vi "Write Frame (iSUB) (SubVI).vi"(5 "Data":T1, 8 "Record":bool, 11 "FILE REF IN":refnum<file>) -> (3 "FILE REF OUT":refnum<file>)   [LabVIEW 2015]
uses:
  Controls (HOST)/Data to Disk Bundle.ctl
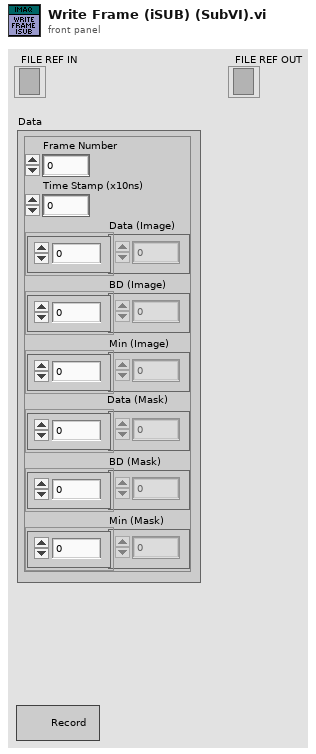
[diagram p1: front panel]
types:
  T1 = typedef "Data to Disk Bundle.ctl" = cluster{"Frame Number":u64, "Time Stamp (x10ns)":u64, "Data (Image)":u64[], "BD (Image)":u8[], "Min (Image)":u8[], "Data (Mask)":u64[], "BD (Mask)":u8[], "Min (Mask)":u8[]}
  T2 = enum16{"big-endian, network order", "native, host order", "little-endian"}
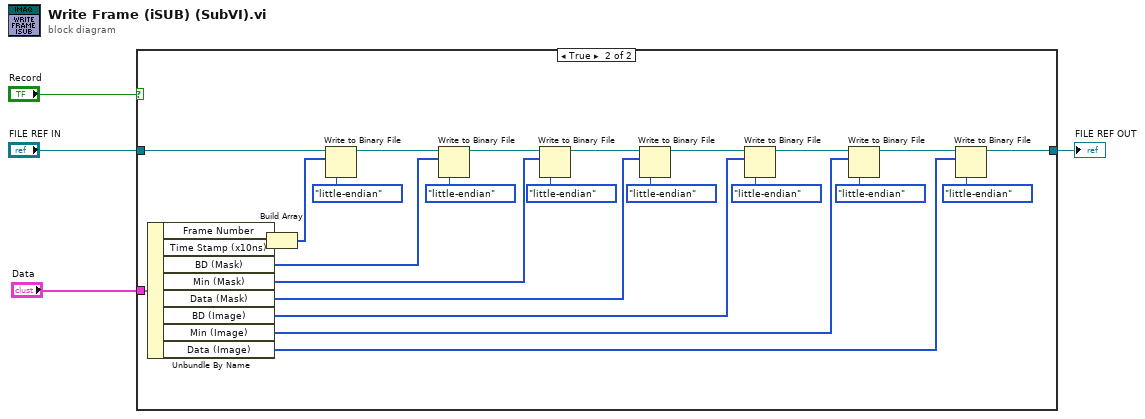
[diagram p0: block diagram]
diagram:
  n1 = case shown="True" "Record" {
    tunnel: [w5 w15] -> w4
    tunnel: "FILE REF IN" -> [w5 w27]
    tunnel: "Data" -> [_ w25]
    frame False {
    }
    frame True {
      n2 = Unbundle By Name(w25) -> ("Frame Number"=w14:u64, "Time Stamp (x10ns)"=w13:u64, "BD (Mask)"=w11:u8[], "Min (Mask)"=w10:u8[], "Data (Mask)"=w9:u64[], "BD (Image)"=w8:u8[], "Min (Image)"=w7:u8[], "Data (Image)"=w6:u64[])
      n3 = Build Array(w14, w13) -> (w12:u64[])
      n4 = Write to Binary File(file (use dialog)=w27, data=w12, 9:T2."little-endian" ("byte order (0:big-endian, network order)")) -> (refnum out=w26:refnum<file>)  [unwired: 3 in, 2 out]
      n5 = Write to Binary File(file (use dialog)=w26, data=w11, 9:T2."little-endian" ("byte order (0:big-endian, network order)")) -> (refnum out=w21:refnum<file>)  [unwired: 3 in, 2 out]
      n6 = Write to Binary File(file (use dialog)=w21, data=w10, 9:T2."little-endian" ("byte order (0:big-endian, network order)")) -> (refnum out=w24:refnum<file>)  [unwired: 3 in, 2 out]
      n7 = Write to Binary File(file (use dialog)=w24, data=w9, 9:T2."little-endian" ("byte order (0:big-endian, network order)")) -> (refnum out=w20:refnum<file>)  [unwired: 3 in, 2 out]
      n8 = Write to Binary File(file (use dialog)=w20, data=w8, 9:T2."little-endian" ("byte order (0:big-endian, network order)")) -> (refnum out=w17:refnum<file>)  [unwired: 3 in, 2 out]
      n9 = Write to Binary File(file (use dialog)=w17, data=w7, 9:T2."little-endian" ("byte order (0:big-endian, network order)")) -> (refnum out=w16:refnum<file>)  [unwired: 3 in, 2 out]
      n10 = Write to Binary File(file (use dialog)=w16, data=w6, 9:T2."little-endian" ("byte order (0:big-endian, network order)")) -> (refnum out=w15:refnum<file>)  [unwired: 3 in, 2 out]
    }
  }
  "FILE REF OUT" <- w4
